vi "Read ADCS.vi"(0 "Sampling Period (ms) (50ms)":i64=50, 1 "Num Samples  to Average (5)":i32=5) -> (6 "ADC Readings (filtered)":T2)   [LabVIEW 2017]
uses:
  <vilib>/Platform/TimedLoop/XDataNode/timing_clust.ctl
  <vilib>/Platform/TimedLoop/XDataNode/nitl_modes.ctl
  <vilib>/Platform/TimedLoop/XDataNode/wakeup.ctl
  <vilib>/myRIO/Instrument Drivers/Onboard IO/AI/typedefs/AI Reference.ctl
  <vilib>/myRIO/Common/Instrument Driver Framework/Utilities/typedefs/myRIO Generic Hardware Reference.ctl
  <vilib>/myRIO/Common/Instrument Driver Framework/Utilities/typedefs/Hardware Version Enum.ctl
  <vilib>/myRIO/Common/Instrument Driver Framework/Utilities/typedefs/myRIO v1.0 Reference.ctl
  <vilib>/myRIO/Common/Instrument Driver Framework/Utilities/typedefs/Generic FPGA Reference.ctl
  <vilib>/myRIO/Common/Instrument Driver Framework/myRIO v1.0/AI/typedefs/AI Channels List.ctl
  <vilib>/myRIO/Common/Instrument Driver Framework/myRIO v1.0/AI/typedefs/AI Channels Enum.ctl
  <vilib>/myRIO/Common/Instrument Driver Framework/Utilities/typedefs/Analog Scaling Constants List.ctl
  <vilib>/myRIO/Common/Instrument Driver Framework/Utilities/typedefs/Analog Scaling Constants.ctl
  <vilib>/userdefined/High Color/nirio_resource_hc.ctl
  <vilib>/myRIO/Common/Instrument Driver Framework/Utilities/vis/Is FPGA Ref Available.vi
  <vilib>/myRIO/Common/Instrument Driver Framework/myRIO v1.0/AI/vis/myRIO v1.1 Open AI.vi
  <vilib>/myRIO/Instrument Drivers/Onboard IO/AI/vis/Read.vi
  <vilib>/myRIO/Common/Instrument Driver Framework/Utilities/vis/Validate Channels.vi
  <vilib>/myRIO/Common/Instrument Driver Framework/myRIO v1.0/AI/vis/myRIO v1.0 Reserve AI.vi
  <vilib>/myRIO/Common/Instrument Driver Framework/myRIO v1.0/AI/vis/myRIO v1.0 Build MUX Configuration AI.vi
  <vilib>/myRIO/Common/Instrument Driver Framework/myRIO v1.0/Resource Manager/vis/myRIO v1.0 Reserve Channel List.vi
  <vilib>/myRIO/Common/Instrument Driver Framework/myRIO v1.0/Resource Manager/vis/myRIO v1.0 Reserve Channel.vi
  <vilib>/myRIO/Common/Instrument Driver Framework/myRIO v1.0/Resource Manager/vis/myRIO v1.0 Unreserve Channel.vi
  <vilib>/myRIO/Common/Instrument Driver Framework/myRIO v1.0/Resource Manager/vis/myRIO v1.0 Build Mutex Name.vi
  <vilib>/Utility/VariantDataType/GetNumericInfo.vi
  <vilib>/Utility/error.llb/Error Cluster From Error Code.vi
  <vilib>/myRIO/Common/Instrument Driver Framework/myRIO v1.0/myRIO v1.1 Open.vi
  <vilib>/myRIO/Common/Instrument Driver Framework/myRIO v1.0/AI/vis/myRIO v1.0 Get Scaling Constants AI.vi
  <vilib>/myRIO/Common/Instrument Driver Framework/Utilities/vis/IO Manager.vi
  <vilib>/myRIO/Common/Instrument Driver Framework/Utilities/vis/Configuration Manager.vi
  <vilib>/myRIO/Common/Instrument Driver Framework/myRIO v1.0/myRIO v1.0 Close.vi
  <vilib>/myRIO/Common/Instrument Driver Framework/myRIO v1.0/AI/vis/myRIO v1.0 Read AI.vi
  <vilib>/platform/TimedLoop/XDataNode/XDataNode.xnode
  <vilib>/myRIO/Express VI/Onboard IO/AI/AI Express VI.xnode
  <vilib>/myRIO/Instrument Drivers/Onboard IO/AI/vis/myRIO AI Open.xnode
  <vilib>/Platform/TimedLoop/XDataNode/XDNodeRunTimeDep.lvlib
  <vilib>/myRIO/Instrument Drivers/Onboard IO/AI/AI.lvlib
panel:
  in  "Rounding Factor (0.001 volts)":T1(ring)
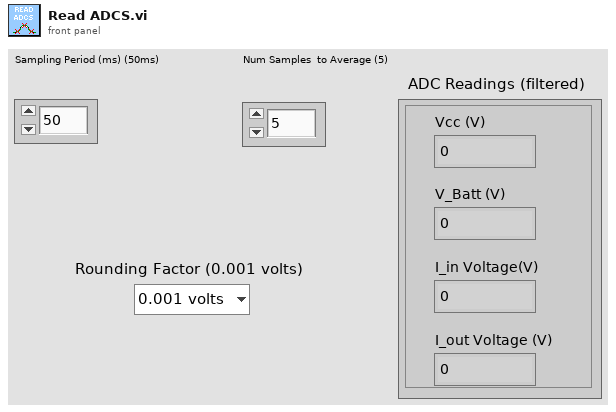
[diagram p1: front panel]
types:
  T1 = enum16{"0.001 volts", "0.01 volts", "0.1 volts", "1 volt"}
  T2 = cluster{"Vcc (V)":dbl, "V_Batt (V)":dbl, "I_in Voltage(V)":dbl, "I_out Voltage (V)":dbl}
  T3 = typedef "XDNodeRunTimeDep.lvlib/timing_clust.ctl" = cluster{"Expected End [f-1]":u64, "Actual End [f-1]":u64, "Finished Late? [f-1]":bool, "Expected End [i-1]":u64, "Actual End [i-1]":u64, "Finished Late? [i-1]":bool, "Expected Start [i]":u64, "Actual Start [i]":u64, "Expected Start [f]":u64, "Actual Start [f]":u64, "Source Name":string, "Structure Name":string, "Period":i64, "Deadline":i64, "Offset":i64, "Start":i64, "Priority":i32, "Timeout":i32, "Mode":T4, "Wakeup Reason":T5, "Error":errorcluster, "Source Type":string, "Secondary Source Type":string, "Global End Time":u64, "Global Start Time":u64, "Frame Duration":u64, "Iteration Duration":u64, "Assigned CPU":i32, "I/O Scan Engine Mode":u32}
  T4 = typedef "XDNodeRunTimeDep.lvlib/nitl_modes.ctl" = enum32{"No Change", "Process missed periods, maintain original phase", "Discard missed periods, maintain original phase", "Process missed periods, ignore original phase", "Discard missed periods, ignore original phase"}
  T5 = typedef "XDNodeRunTimeDep.lvlib/wakeup.ctl" = enum32{"Normal", "Aborted", "Asynchronous wakeup", "Timing source error", "Timed loop error", "Timeout"}
  T6 = typedef "AI.lvlib/AI Reference.ctl" = cluster{"myRIO Reference":T7, "AI Channels List":T11, "AI Scaling Constants List":T13}
  T7 = typedef "myRIO Generic Hardware Reference.ctl" = cluster{"myRIO Model":T8, "myRIO Hardware Reference":T9}
  T8 = typedef "Hardware Version Enum.ctl" = enum16{"Unknown", "myRIO-1900", "myRIO-1950", "roboRIO", "NI ELVIS RIO CM"}
  T9 = typedef "myRIO v1.0 Reference.ctl" = cluster{"Generic FPGA Reference":T10, "Allow multiple opens":bool}
  T10 = typedef "Generic FPGA Reference.ctl" = refnum<k20>
  T11 = typedef "AI Channels List.ctl" = T12[]
  T12 = typedef "AI Channels Enum.ctl" = enum16{"Not Connected", "AudioIn/Left", "AudioIn/Right", "C/AI0", "C/AI1", "A/AI0", "A/AI1", "A/AI2", "A/AI3", "B/AI0", "B/AI1", "B/AI2", "B/AI3", "AI/AI0", "AI/AI1", "AI/AI2", "AI/AI3"}
  T13 = typedef "Analog Scaling Constants List.ctl" = T14[]
  T14 = typedef "Analog Scaling Constants.ctl" = cluster{"LSB Weight (Volts)":dbl, "Offset (Volts)":dbl, "Signed?":bool}
  T15 = typedef "nirio_resource_hc.ctl" = tag
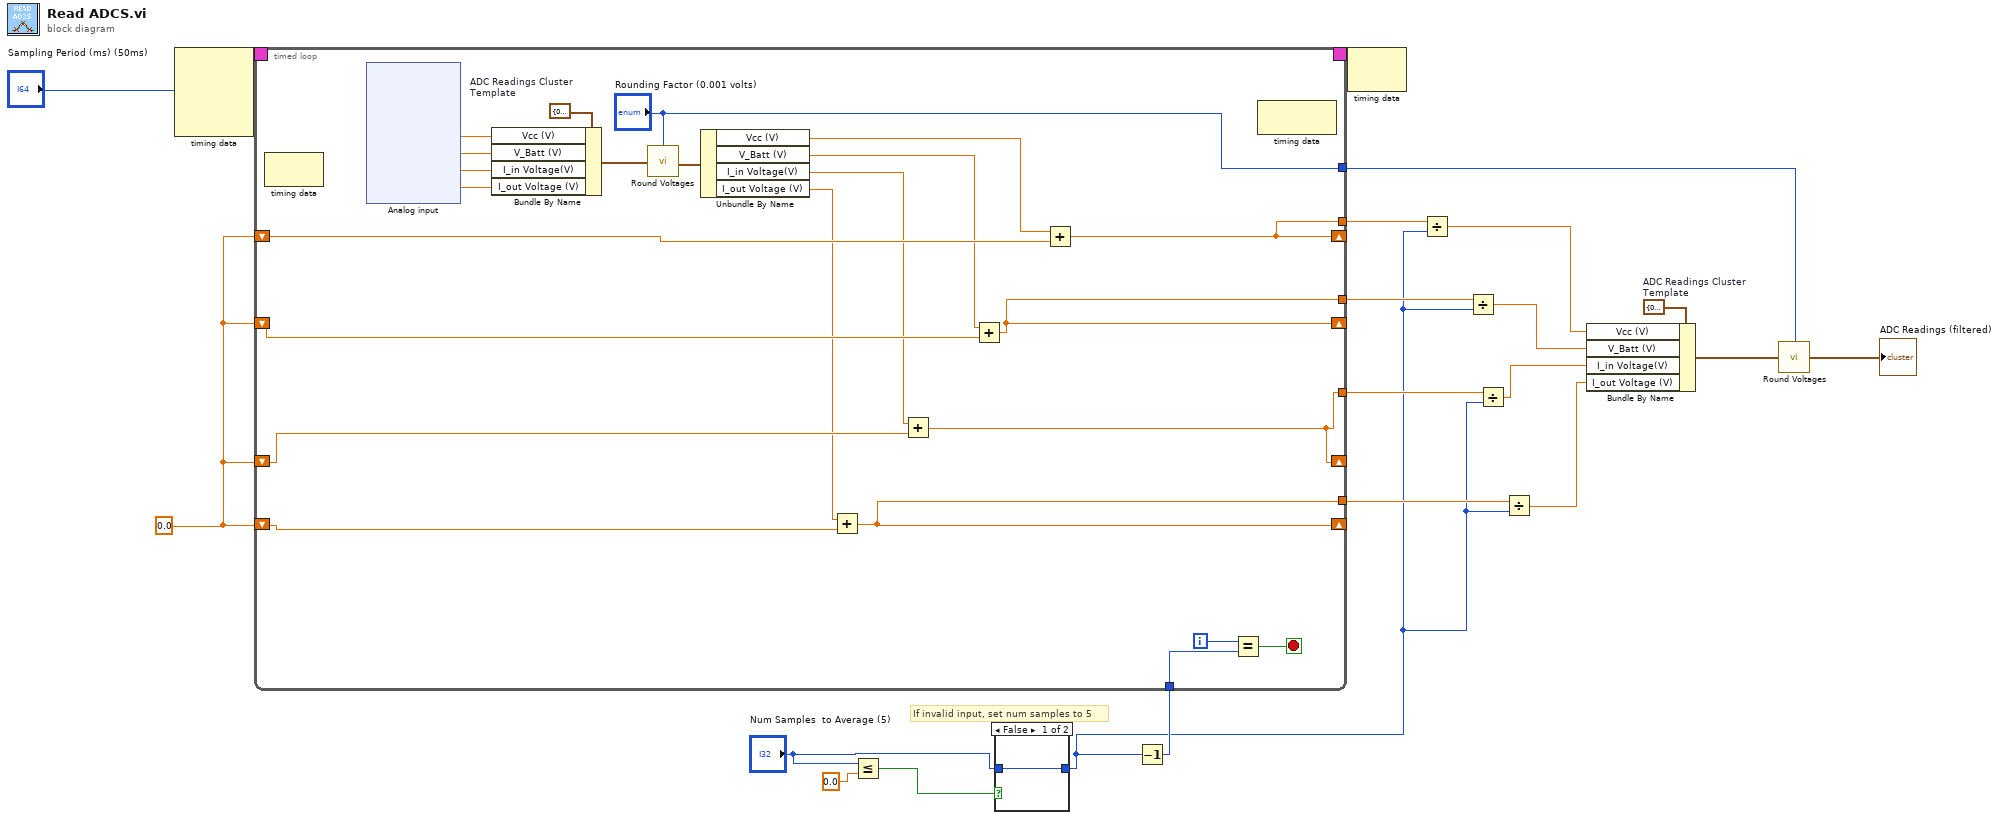
[diagram p0: block diagram]
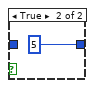
[diagram p2: hidden frame]
diagram:
  w13 = T2 {"Vcc (V)"=0.0, "V_Batt (V)"=0.0, "I_in Voltage(V)"=0.0, "I_out Voltage (V)"=0.0}  # ADC Readings Cluster Template
  w7 = 0.0
  # "If invalid input, set num samples to 5"
  n1 = node-c288("Sampling Period (ms) (50ms)") -> (w21:T3)  [unwired: 3 in]
  n2 = Less Or Equal?(x="Num Samples  to Average (5)", y=0.0) -> (x <= y?=w17:bool)
  n3 = case shown="False" w17 {
    tunnel: "Num Samples  to Average (5)" -> [w22 _]
    tunnel: [w22 5] -> w5
    frame False {
    }
    frame True {
    }
  }
  n4 = Decrement(x=w5) -> (x-1=w19:i32)
  n5 = timed-loop {
    timing: w21 -> [_]
    timing-out: [_] -> w20
    tunnel: w19 -> [w44]
    shift-right: [w42] -> _
    shift-left: w7 -> [w43]
    tunnel: [w42] -> w14
    shift-right: [w40] -> _
    shift-left: w7 -> [w41]
    tunnel: [w40] -> w12
    shift-right: [w38] -> _
    shift-left: w7 -> [w39]
    tunnel: [w38] -> w9
    shift-right: [w36] -> _
    shift-left: w7 -> [w37]
    tunnel: [w36] -> w6
    tunnel: ["Rounding Factor (0.001 volts)"] -> w1
    i -> [w46]
    stop <- w45 stop-if-true
    w35 = T2 {"Vcc (V)"=0.0, "V_Batt (V)"=0.0, "I_in Voltage(V)"=0.0, "I_out Voltage (V)"=0.0}  # ADC Readings Cluster Template
    n6 = node-c288() -> ()  [unwired: 1 in, 1 out]
    n7 = xnode "Analog input"() -> ("Vcc (A/AI0 (Pin 3))"=w31:dbl, "Batt+ (A/AI1 (Pin 5))"=w32:dbl, "Iin Voltage (A/AI2 (Pin 7))"=w33:dbl, "Iout Voltage (A/AI3 (Pin 9))"=w34:dbl)  [unwired: 1 in, 1 out]
    n8 = Bundle By Name(cluster=w35, "Vcc (V)"=w31, "V_Batt (V)"=w32, "I_in Voltage(V)"=w33, "I_out Voltage (V)"=w34) -> (w30:T2)
    n9 = call "Round Voltages.vi"("Rouding Factor (0.001 volts)"="Rounding Factor (0.001 volts)", "ADC Readings (rounded)"=w30) -> ("ADC Readings (rounded)"=w29:T2)  [unwired: 13 in]
    n10 = Unbundle By Name(w29) -> ("Vcc (V)"=w25:dbl, "V_Batt (V)"=w26:dbl, "I_in Voltage(V)"=w27:dbl, "I_out Voltage (V)"=w28:dbl)
    n11 = Add(x=w28, y=w43) -> (x+y=w42:dbl)
    n12 = Add(x=w27, y=w41) -> (x+y=w40:dbl)
    n13 = Add(x=w26, y=w39) -> (x+y=w38:dbl)
    n14 = Add(x=w25, y=w37) -> (x+y=w36:dbl)
    n15 = Equal?(x=w46, y=w44) -> (x = y?=w45:bool)
    n16 = node-c288() -> ()  [unwired: 1 in, 1 out]
  }
  n17 = node-c288(w20) -> ()  [unwired: 1 out]
  n18 = Divide(x=w6, y=w5) -> (x/y=w4:dbl)
  n19 = Divide(x=w9, y=w5) -> (x/y=w8:dbl)
  n20 = Divide(x=w12, y=w5) -> (x/y=w10:dbl)
  n21 = Divide(x=w14, y=w5) -> (x/y=w11:dbl)
  n22 = Bundle By Name(cluster=w13, "Vcc (V)"=w4, "V_Batt (V)"=w8, "I_in Voltage(V)"=w10, "I_out Voltage (V)"=w11) -> (w3:T2)
  n23 = call "Round Voltages.vi"("Rouding Factor (0.001 volts)"=w1, "ADC Readings (rounded)"=w3) -> ("ADC Readings (rounded)"=→"ADC Readings (filtered)":T2)  [unwired: 13 in]
